vi "New File.vi"(8 "error in":errorcluster, 11 "File in":refnum<class "File.lvclass">) -> (0 "error out":errorcluster, 3 "File out":refnum<class "File.lvclass">)   [LabVIEW 2013, in "File.lvclass"]
uses:
  File.lvclass
  File.lvclass/File.ctl
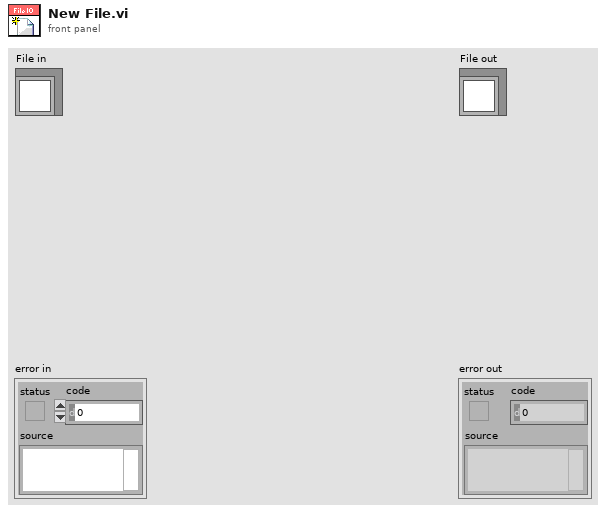
[diagram p1: front panel]
types:
  T1 = enum16{"open", "replace", "create", "open or create", "replace or create", "replace or create with confirmation"}
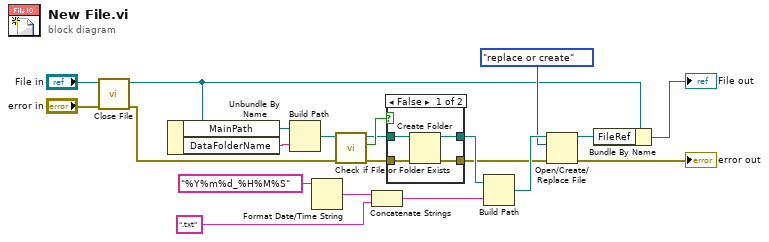
[diagram p0: block diagram]
diagram:
  n1 = call-dynamic "Close File.vi"("error in"="error in", "File in"="File in") -> ("error out"=w2:errorcluster, "File out"=w5:refnum<class "File.lvclass">)  [unwired: 8 in]
  n2 = Unbundle By Name(w5) -> ("MainPath"=w20:path, "DataFolderName"=w19:string)
  n3 = Build Path(base path=w20, name or relative path=w19) -> (appended path=w14:path)
  n4 = Format Date/Time String(time format string (%c)="%Y%m%d_%H%M%S") -> (date/time string=w17:string)  [unwired: 2 in]
  n5 = call <vilib>:"Check if File or Folder Exists.vi"("error in (no error)"=w2, "path"=w14) -> ("error out"=w11:errorcluster, "file or folder exists?"=w13:bool, "dup path"=w12:path)  [unwired: 7 in]
  n6 = Concatenate Strings(w17, ".txt" ("string")) -> (w15:string)
  n7 = case shown="False" w13 {
    tunnel: w12 -> [w25 w27]
    tunnel: [w24 w27] -> w10
    tunnel: [w23 w26] -> w7
    tunnel: w11 -> [w22 w26]
    frame False {
      n8 = Create Folder(path (use dialog)=w25, error in=w22) -> (created path=w24:path, error out=w23:errorcluster)  [unwired: 1 in, 1 out]
    }
    frame True {
    }
  }
  n9 = Build Path(base path=w10, name or relative path=w15) -> (appended path=w9:path)
  n10 = Open/Create/Replace File(file path (use dialog)=w9, error in=w7, operation (0:open)=T1."replace or create") -> (refnum out=w4:refnum<file>, error out=→"error out":errorcluster)  [unwired: 3 in, 1 out]
  n11 = Bundle By Name(cluster=w5, "FileRef"=w4) -> (→"File out":refnum<class "File.lvclass">)
